vi "Init.vi"(9 "Event jettl":refnum<class "Event jettl.lvclass">, 10 "Alias":string) -> (3 "Event Create Msg Strategy out":refnum<class "Event Create Msg Strategy.lvclass">)   [LabVIEW 2021, in "jettl.lvlib" / "Event Create.lvlib" / "Event Create Msg Strategy.lvclass"]
uses:
  Event Create Msg Strategy.lvclass
  Event jettl/Event jettl.lvclass
  Event Create Msg Strategy.lvclass/Event Create Msg Strategy.ctl
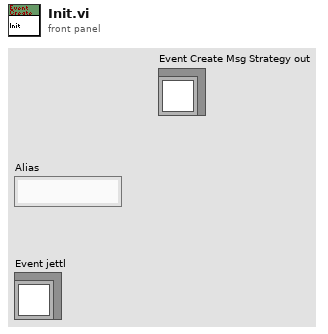
[diagram p1: front panel]
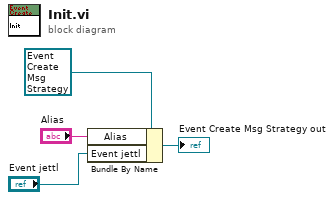
[diagram p0: block diagram]
diagram:
  n1 = Bundle By Name(cluster=refnum<class "Event Create Msg Strategy.lvclass"> refnum ("Event Create Msg out"), "Alias"="Alias", "Event jettl"="Event jettl") -> (→"Event Create Msg Strategy out":refnum<class "Event Create Msg Strategy.lvclass">)
